vi "公式波形发生器.vi"() -> ()   [LabVIEW 2012]
uses:
  <vilib>/gmath/NI_Gmath.lvlib
panel:
  in  "formula":string="10*sin(x)*cos(2*x)+rand(-1)" caption="公式"
  in  "end":dbl=12.56 caption="结束" format="%.2f"
  in  "start":dbl caption="开始" format="%.2f"
  in  "number of points":u32=100 caption="点数"
  in  "停止":bool
  out "波形图":dbl[](graph)=[0.4253531630032392, 1.8404521755843644, 2.908269634134502, 3.213013458518826, 2.87155469325695, 1.980707871431694, 1.2777188029823672, -0.9240613157547477, -2.968973826733148, -5.575682876912691, -7.069987278362677, -8.93972175392823, -9.068584427121875, -8.906970413469462, -8.997248806384679, -7.659260234533236, -4.925706723538203, -3.2508065141738514, -1.320723232341108, 0.5728374113638073, 1.8534292538810084, 3.1649508582004056, 3.678919644538743, 2.6804576898634007, 2.0990259754956484, 0.9291219221653082, -1.0317069575995355, -1.5649063541193187, -1.7278708718446398, -2.442365273896862, -1.0361019942844882, -0.17669202823953978, 2.034580265831585, 4.266284455534657, 6.28872443275799, 8.497611576178828, 9.990612840390142, 9.922154358954977, 10.246964540260972, 9.473523059304188, 7.9126375803210145, 5.849076243948188, 3.874169832924167, 1.7726631002802258, 0.2876204762371628, -1.3826101608523496, -2.4760184259567453, -2.4766065908389017, -1.32942849538584, -1.2123727004591798, 0.15681903303062716, 1.238726906834595, 2.256311951766767, 2.85578378576102, 3.1056957758005446, 2.1766522344035275, 1.2115429031795364, -1.0997123213619626, -3.096653377160999, -5.644469510319574, -7.57978586600016, -8.351376763774665, -9.44879625015377, -9.539208547336187, -8.974892171857443, -7.718135976769457, -5.261680840022079, -3.095267333271885, -1.2903616848056991, 0.6861020389793322, 2.0135981169689408, 2.83990744960959, 3.3888406910198676, 2.881762130622235, 1.3716136801054786, 0.2880282619740062, -0.9027650831381395, -1.293856314607487, -1.8444099292849816, -2.4608464435024517, -1.8195956116984886, -0.07600289349523831, 2.026231802134801, 4.48570816737399, 5.903356642926397, 8.294338725280298, 9.653244012904286, 10.824393256225497, 9.985449414499392, 9.376638575839575, 8.708528065125373, 6.685081665771653, 3.9819361395672943, 1.977978240744965, 0.3926125223914356, -0.9150083867453862, -1.7388436553482325, -1.8500256032520832, -1.4951531969966563, -0.6707765736908413]
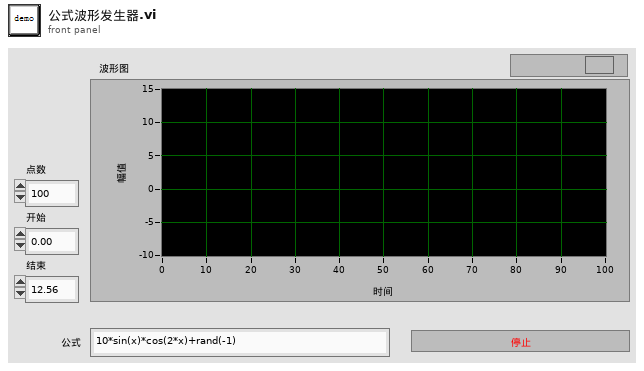
[diagram p1: front panel]
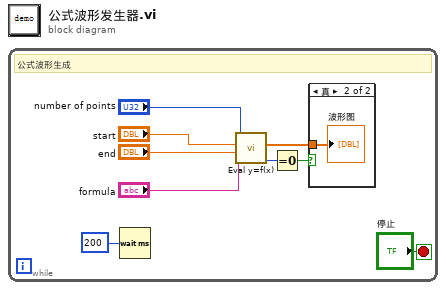
[diagram p0: block diagram]
diagram:
  n1 = while {
    stop <- "停止" stop-if-true
    # "公式波形生成"
    n2 = Wait (ms)(milliseconds to wait=u32 200 ("等待时间（毫秒）")) -> ()  [unwired: 1 out]
    n3 = call <vilib>:"Eval y=f(x).vi"("formula"="formula", "end"="end", "start"="start", "number of points"="number of points") -> ("error"=w3:i32, "Y Values"=w2:dbl[])  [unwired: 2 out]
    n4 = Equal To 0?(x=w3) -> (x = 0?=w4:bool)
    n5 = case shown="真" w4 {
      tunnel: w2 -> [_ w10]
      frame False {
      }
      frame True {
        "波形图" <- w10
      }
    }
  }
